vi "OnDataChange.vi"(0 "GRMActor in":refnum<class "GeneralRMActor.lvclass">, 1 "DataExchange":T1, 3 "error in (no error)":errorcluster) -> (7 "GRMActor out":refnum<class "GeneralRMActor.lvclass">, 10 "error out":errorcluster)   [LabVIEW 2020, in "GeneralRMActor.lvlib" / "GeneralRMActor.lvclass"]
uses:
  GeneralRMActor.lvclass
  Device/Device/DataExchange.ctl
  Interface/DataListener Messages/OnDataChange Msg/OnDataChange Msg.lvclass/OnDataChange Msg.ctl
  <vilib>/ActorFramework/Message Enqueuer/Message Enqueuer.lvclass/Message Enqueuer.ctl
  <vilib>/ActorFramework/Message Enqueuer/Message Enqueuer.lvclass
  GeneralRMActor.lvclass/GeneralRMActor.ctl
  <vilib>/ActorFramework/Message Enqueuer/Enqueue.vi
  Interface/DataListener Messages/OnDataChange Msg/OnDataChange Msg.lvclass
  C:/Program Files/National Instruments/LabVIEW 2020/vi.lib/ActorFramework/Message/Message.lvclass
  <vilib>/ActorFramework/Message Priority Queue/Priority Enqueue.vi
  Interface/DataListener/DataListener.lvclass
panel:
  out "error out 2":errorcluster
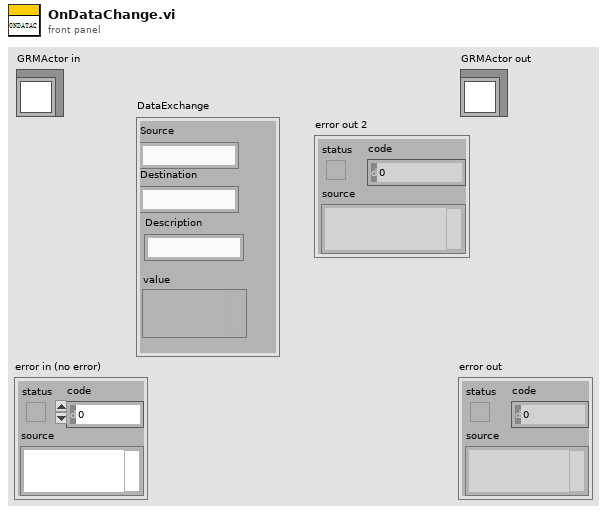
[diagram p1: front panel]
types:
  T1 = typedef "DataListener.lvclass/DataExchange.ctl" = cluster{"Source":string, "Destination":string, "Description":string, "value":variant}
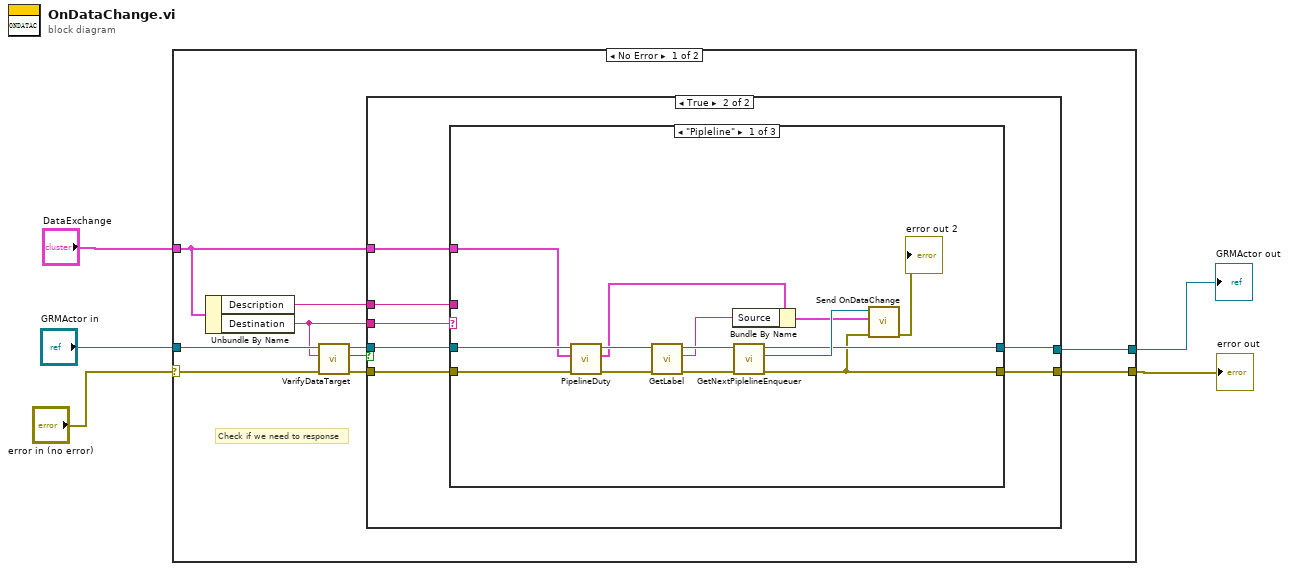
[diagram p0: block diagram]
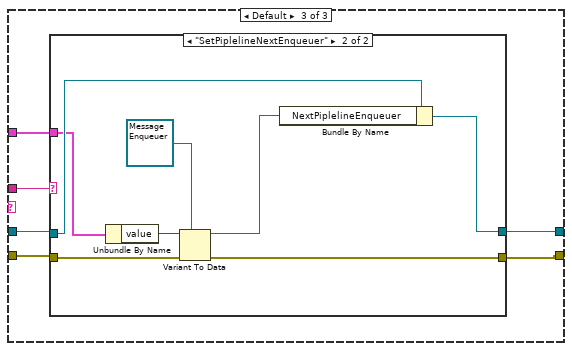
[diagram p4: hidden frame]
diagram:
  n1 = case shown="No Error" "error in (no error)" {
    selector: "error in (no error)" -> [w13 w58]
    tunnel: [w14 w58] -> w4
    tunnel: "GRMActor in" -> [w11 w57]
    tunnel: [w15 w57] -> w3
    tunnel: "DataExchange" -> [w9 _]
    frame No Error {
      # "Check if we need to response"
      n2 = Unbundle By Name(w9) -> ("Description"=w7:string, "Destination"=w6:string)
      n3 = call-dynamic "VarifyDataTarget.vi"("error in (no error)"=w13, "Destination"=w6, "GRMActor in"=w11) -> ("error out"=w12:errorcluster, "Response?"=w8:bool, "GRMActor out"=w10:refnum<class "GeneralRMActor.lvclass">)  [unwired: 6 in]
      n4 = case shown="True" w8 {
        tunnel: [w17 w24] -> w15
        tunnel: w10 -> [w17 w23]
        tunnel: [w16 w21] -> w14
        tunnel: w12 -> [w16 w22]
        tunnel: w9 -> [_ w20]
        tunnel: w7 -> [_ w19]
        tunnel: w6 -> [_ w18]
        frame False {
        }
        frame True {
          n5 = case shown="\"Pipleline\"" w18 {
            tunnel: [w27 w39 w46] -> w24
            tunnel: w23 -> [w29 w39 w45]
            tunnel: w22 -> [w30 w40 w44]
            tunnel: [w26 w40 w43] -> w21
            tunnel: w20 -> [w28 _ w42]
            tunnel: w19 -> [_ _ w41]
            frame "Pipleline" {
              n6 = call-dynamic "PipelineDuty.vi"("error in (no error)"=w30, "DataExchange"=w28, "GRMActor in"=w29) -> ("error out"=w38:errorcluster, "DataExchange 2"=w32:T1, "GRMActor out"=w36:refnum<class "GeneralRMActor.lvclass">)  [unwired: 6 in]
              n7 = call-dynamic "GetLabel.vi"("error in (no error)"=w38, "GRMActor in"=w36) -> ("error out"=w37:errorcluster, "Label"=w31:string, "GRMActor out"=w35:refnum<class "GeneralRMActor.lvclass">)  [unwired: 7 in]
              n8 = Bundle By Name(cluster=w32, "Source"=w31) -> (w33:T1)
              n9 = call-dynamic "GetNextPiplelineEnqueuer.vi"("error in (no error)"=w37, "GRMActor in"=w35) -> ("error out"=w26:errorcluster, "NextPiplelineEnqueuer"=w34:refnum<class "Message Enqueuer.lvclass">, "GRMActor out"=w27:refnum<class "GeneralRMActor.lvclass">)  [unwired: 7 in]
              n10 = call "Send OnDataChange.vi"("error in (no error)"=w26, "DataExchange"=w33, "Message Enqueuer"=w34) -> ("error out"=→"error out 2":errorcluster)  [unwired: 7 in, 1 out]
            }
            frame "Broadcast" {
            }
            frame Default {
              n11 = case shown="\"SetPiplelineNextEnqueuer\"" w41 {
                tunnel: [w48 w53] -> w46
                tunnel: w45 -> [w48 w54]
                tunnel: [w47 w55] -> w43
                tunnel: w44 -> [w47 w56]
                tunnel: w42 -> [_ w52]
                frame Default {
                }
                frame "SetPiplelineNextEnqueuer" {
                  n12 = Unbundle By Name(w52) -> ("value"=w51:variant)
                  n13 = Variant To Data(error in=w56, type=refnum<class "Message Enqueuer.lvclass"> refnum ("Enqueuer"), Variant=w51) -> (data=w49:refnum<class "Message Enqueuer.lvclass">, error out=w55:errorcluster)
                  n14 = Bundle By Name(cluster=w54, "NextPiplelineEnqueuer"=w49) -> (w53:refnum<class "GeneralRMActor.lvclass">)
                }
              }
            }
          }
        }
      }
    }
    frame Error {
    }
  }
  "error out" <- w4
  "GRMActor out" <- w3
